vi "HumanSetAbsTrajEndPosition.vi"(9 "AbsTrajEndPose_Orient_Deg":dbl, 10 "AbsTrajEndPose_Y_Ft":dbl=13.0, 11 "AbsTrajEndPose_X_Ft":dbl=10.0) -> ()   [LabVIEW 2023]
doc: "Set the desired end position for teleop execute absolute trajectory."
uses:
  <vilib>/Rock Robotics/WPI/ThirdParty/JAS_Junk/TrajLib/Rotation2d_CreateAngle.vi
  <vilib>/Rock Robotics/WPI/ThirdParty/JAS_Junk/TrajLib/Translation2d_Create.vi
  HumanGlobal.vi
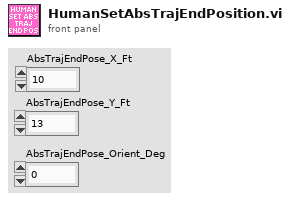
[diagram p1: front panel]
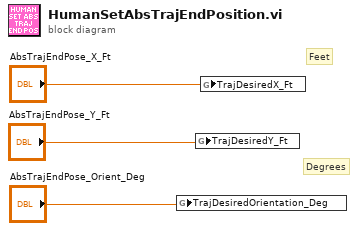
[diagram p0: block diagram]
diagram:
  # "Degrees"
  # "Feet"
  n1 = global write "HumanGlobal.vi" "TrajDesiredOrientation_Deg"("AbsTrajEndPose_Orient_Deg") -> ()
  n2 = global write "HumanGlobal.vi" "TrajDesiredY_Ft"("AbsTrajEndPose_Y_Ft") -> ()
  n3 = global write "HumanGlobal.vi" "TrajDesiredX_Ft"("AbsTrajEndPose_X_Ft") -> ()
